vi "PVCAM_GetLatestFrame.vi"(7 "error in (no error)":errorcluster, 10 "hCam":i16) -> (0 "error out":errorcluster, 2 "return":i16, 3 "frame ptr":u64)   [LabVIEW 2021]
uses:
  pvcam64.dll
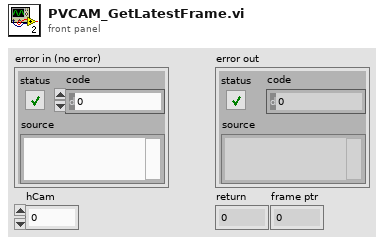
[diagram p1: front panel]
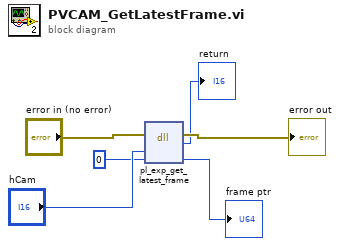
[diagram p0: block diagram]
diagram:
  n1 = dll-call lib="pvcam64.dll" fn="pl_exp_get_latest_frame"(error in="error in (no error)", "hCam"="hCam", "frame ptr"=u64 0) -> (error out=→"error out":errorcluster, "return type"=→"return":i16, "frame ptr"=→"frame ptr":u64)  [unwired: 3 in, 1 out]
